vi "Predet_Ignite.vi"() -> (0 "Digital Waveform Graph":digitalwaveform[](graph), 3 "Error Out":errorcluster)   [LabVIEW 2017]
uses:
  <vilib>/DAQmx/write.llb/DAQmx Write (Digital 1D Wfm NChan NSamp).vi
  <vilib>/DAQmx/create/channels.llb/DAQmx Create Channel (DO-Digital Output).vi
  <vilib>/DAQmx/configure/timing.llb/DAQmx Timing (Sample Clock).vi
  <vilib>/Waveform/DTblOps.llb/DTbl Boolean Array to Digital.vi
  <vilib>/Waveform/DWDTOps.llb/DWDT Uncompress Digital.vi
  <vilib>/DAQmx/miscellaneous.llb/DAQmx Fill In Error Info.vi
  <resource>/objmgr/daqmx.rc
panel:
  in  "error in 2":errorcluster caption="error in"
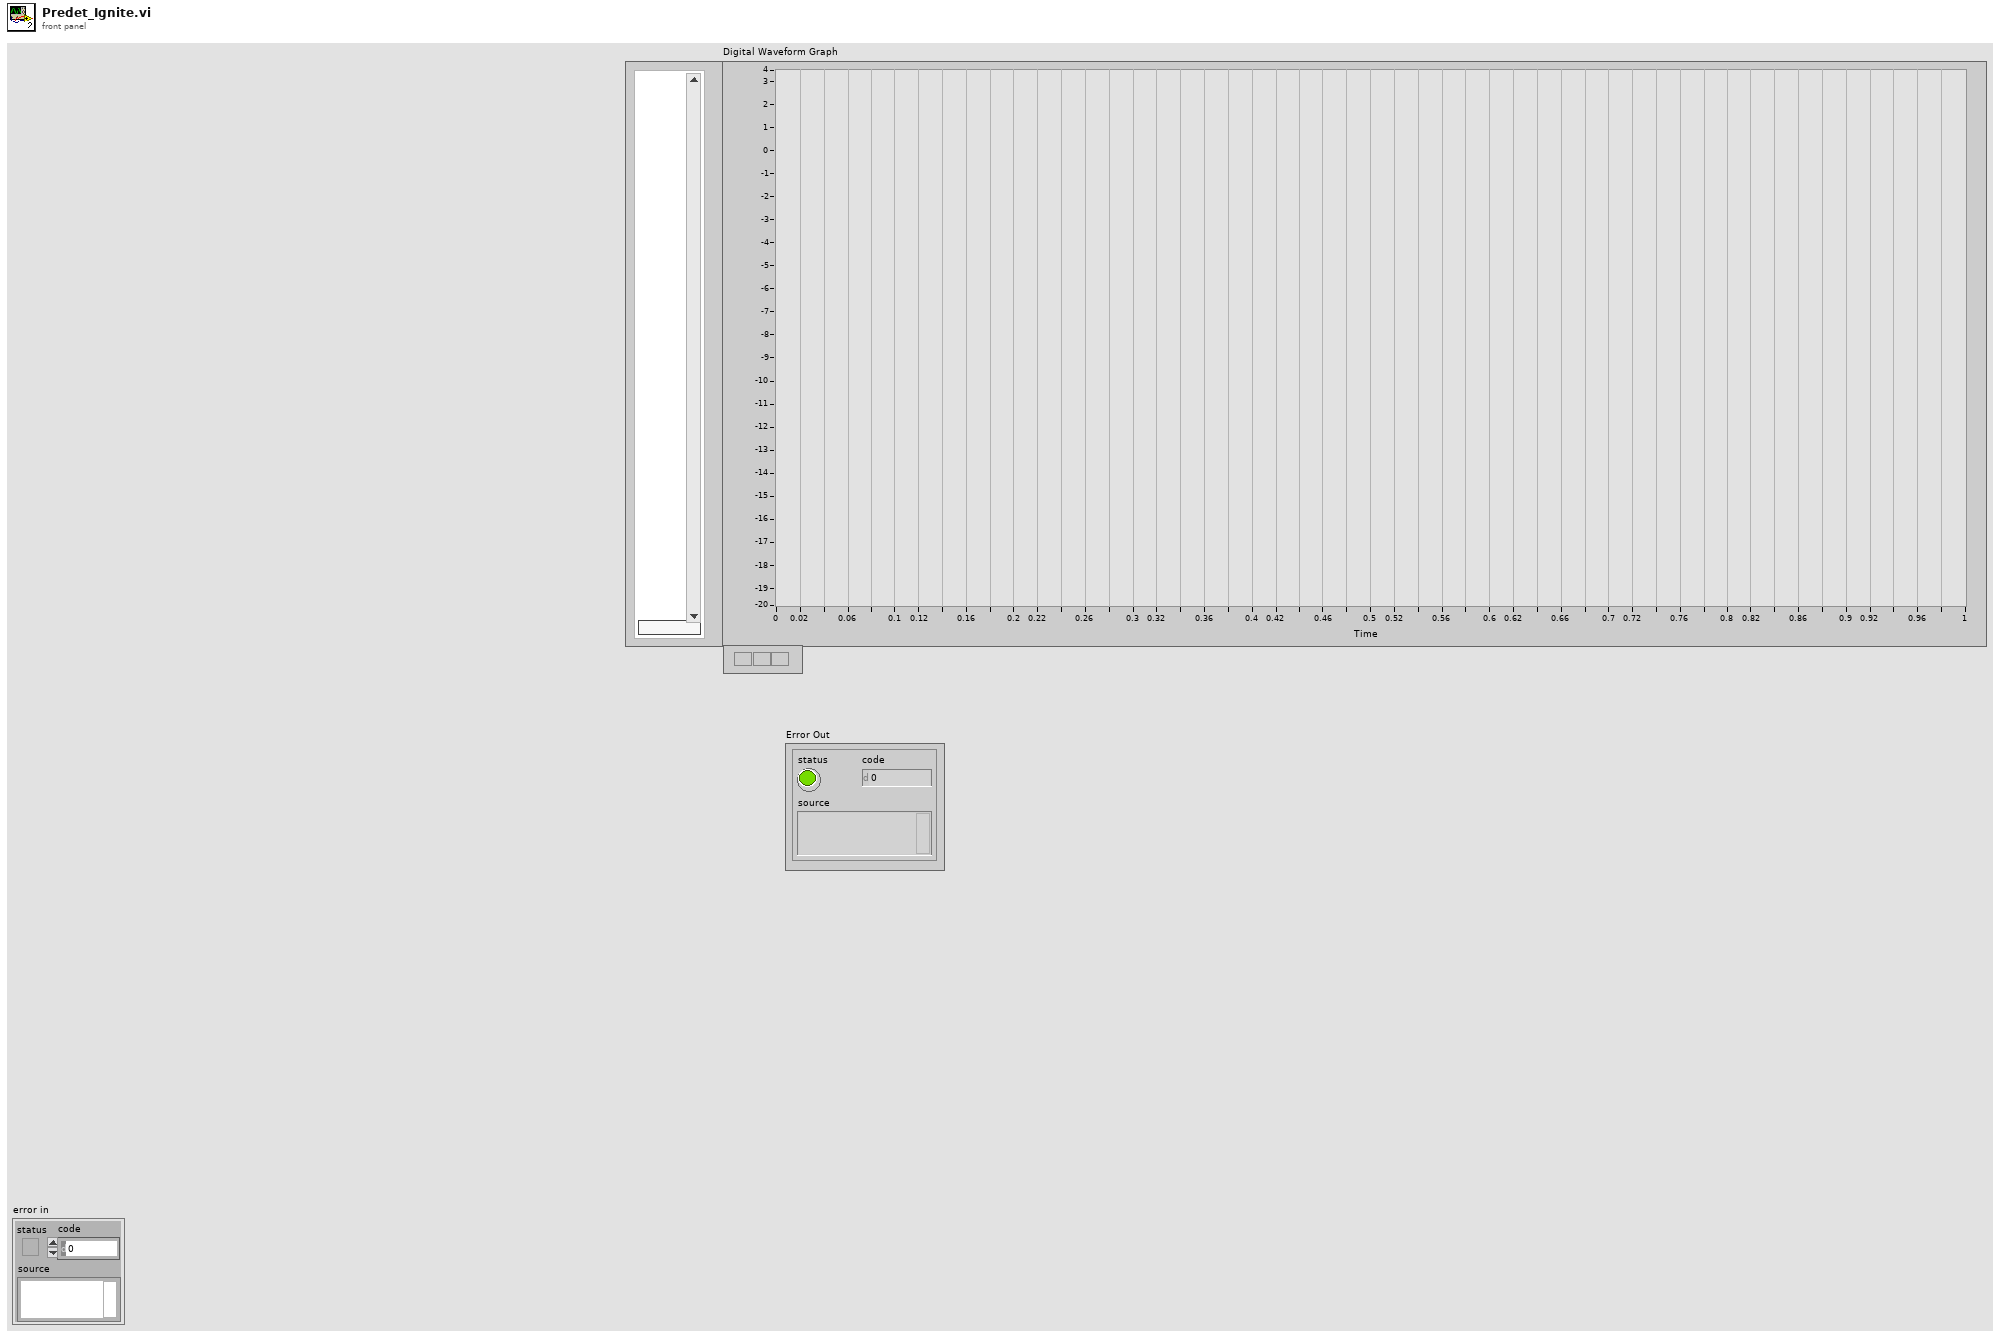
[diagram p1: front panel]
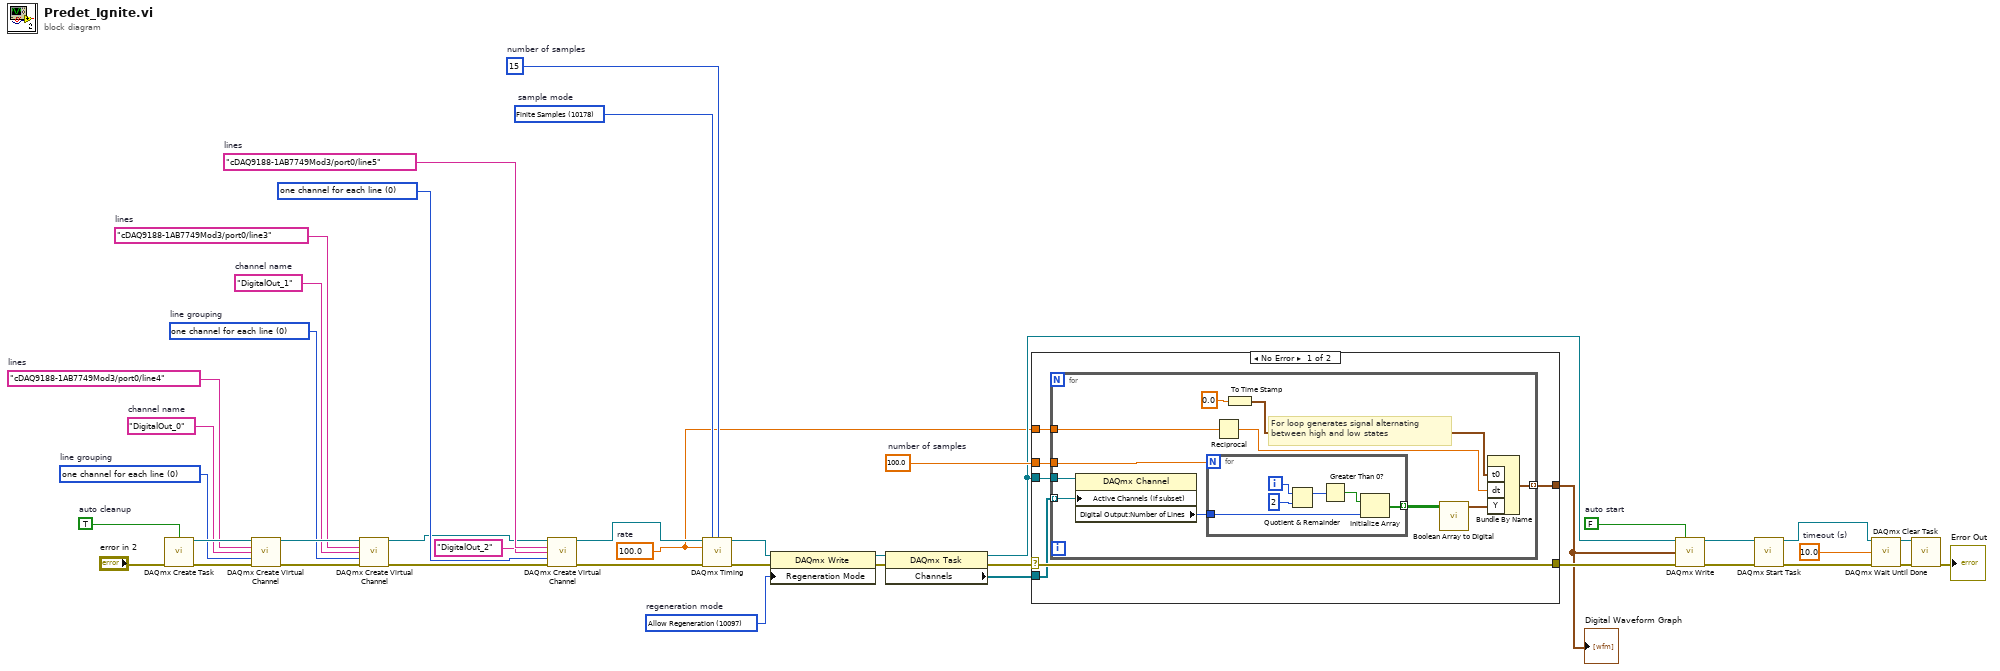
[diagram p0: block diagram]
diagram:
  w6 = "cDAQ9188-1AB7749Mod3/port0/line5"  # lines
  w7 = 0 items=["one channel for each line", "one channel for all lines"] ("line grouping")
  w13 = 10097 items=["Allow Regeneration"=10097, "Do Not Allow Regeneration"=10158]  # regeneration mode
  w15 = 10178 items=["Finite Samples"=10178, "Continuous Samples"=10123, "Hardware Timed Single Point"=12522]  # sample mode
  w16 = 15  # number of samples
  w1 = 100.0  # rate
  w19 = 0 items=["one channel for each line", "one channel for all lines"]  # line grouping
  w18 = "DigitalOut_1"  # channel name
  w20 = "cDAQ9188-1AB7749Mod3/port0/line3"  # lines
  w24 = 0 items=["one channel for each line", "one channel for all lines"]  # line grouping
  w23 = "DigitalOut_0"  # channel name
  w25 = "cDAQ9188-1AB7749Mod3/port0/line4"  # lines
  w27 = TRUE  # auto cleanup
  w35 = 10.0  # timeout (s)
  w32 = 100.0  # number of samples
  w42 = FALSE  # auto start
  n1 = call <vilib>:"DAQmx Create Task.vi"("auto cleanup"=w27, "error in"="error in 2") -> ("task out"=w26:refnum<k21>, "error out"=w28:errorcluster)  [unwired: 12 in]
  n2 = call-poly <vilib>:"DAQmx Create Virtual Channel.vi"("task in"=w26, "lines"=w25, "name to assign"=w23, "line grouping"=w24, "error in"=w28) -> ("task out"=w21:refnum<k21>, "error out"=w22:errorcluster)  [unwired: 9 in]
  n3 = call-poly <vilib>:"DAQmx Create Virtual Channel.vi"("task in"=w21, "lines"=w20, "name to assign"=w18, "line grouping"=w19, "error in"=w22) -> ("task out"=w4:refnum<k21>, "error out"=w9:errorcluster)  [unwired: 9 in]
  n4 = call-poly <vilib>:"DAQmx Create Virtual Channel.vi"("task in"=w4, "lines"=w6, "name to assign"="DigitalOut_2", "line grouping"=w7, "error in"=w9) -> ("task out"=w8:refnum<k21>, "error out"=w10:errorcluster)  [unwired: 9 in]
  n5 = call-poly <vilib>:"DAQmx Timing.vi"("task/channels in"=w8, "sample mode"=w15, "samples per channel"=w16, "rate"=w1, "error in"=w10) -> ("task out"=w14:refnum<k21>, "error out"=w17:errorcluster)  [unwired: 9 in]
  n6 = property class="DAQmx Write"(reference=w14, error in=w17, "Regeneration Mode"=w13) -> (reference out=w12:refnum<k21>, error out=w11:errorcluster)
  n7 = property class="DAQmx Task"(reference=w12, error in=w11) -> (reference out=w30:refnum<k21>, error out=w33:errorcluster, "Channels"=w34:refnum<k21>[])
  n8 = case shown="No Error" w33 {
    selector: w33 -> [w46 w66]
    tunnel: w1 -> [w48 _]
    tunnel: [w47 _] -> w3
    tunnel: [w46 w66] -> w31
    tunnel: w32 -> [w45 _]
    tunnel: w34 -> [w44 _]
    tunnel: w30 -> [w43 _]
    frame No Error {
      n9 = for {
        tunnel: w48 -> [w59]
        tunnel: [w54] -> w47 mode=indexing
        tunnel: w45 -> [w53]
        tunnel: w44 -> [w51] mode=indexing
        tunnel: w43 -> [w49]
        # "For loop generates signal alternating\nbetween high and low states"
        n10 = property class="DAQmx Channel"(reference=w49, "Active Channels (if subset)"=w51) -> ("Digital Output:Number of Lines"=w50:u32)  [unwired: 1 in, 2 out]
        n11 = for {
          N: w53 -> [_]
          tunnel: [w60] -> w52 mode=indexing
          tunnel: w50 -> [w61]
          i -> [w65]
          n12 = Quotient & Remainder(x=w65, y=2) -> (x-y*floor(x/y)=w63:i32)  [unwired: 1 out]
          n13 = Greater Than 0?(x=w63) -> (x > 0?=w62:bool)
          n14 = Initialize Array(w62, w61) -> (w60:bool[])
        }
        n15 = Reciprocal(x=w59) -> (1/x=w55:dbl)
        n16 = To Time Stamp(1:0.0) -> (0:w57:timestamp)
        n17 = call-poly <vilib>:"Boolean Array to Digital.vi"("boolean array"=w52) -> ("digital data"=w56:digitaldata)  [unwired: 3 in, 7 out]
        n18 = Bundle By Name("t0"=w57, "dt"=w55, "Y"=w56) -> (w54:digitalwaveform)  [unwired: 1 out]
      }
    }
    frame Error {
    }
  }
  "Digital Waveform Graph" <- w3
  n19 = call-poly <vilib>:"DAQmx Write.vi"("task/channels in"=w30, "auto start"=w42, "data"=w3, "error in"=w31) -> ("task out"=w38:refnum<k21>, "error out"=w37:errorcluster)  [unwired: 9 in, 1 out]
  n20 = call <vilib>:"DAQmx Start Task.vi"("task/channels in"=w38, "error in"=w37) -> ("task out"=w41:refnum<k21>, "error out"=w40:errorcluster)  [unwired: 12 in]
  n21 = call <vilib>:"DAQmx Wait Until Done.vi"("task/channels in"=w41, "timeout (sec)"=w35, "error in"=w40) -> ("task out"=w36:refnum<k21>, "error out"=w39:errorcluster)  [unwired: 11 in]
  n22 = call <vilib>:"DAQmx Clear Task.vi"("task in"=w36, "error in"=w39) -> ("error out"=→"Error Out":errorcluster)  [unwired: 13 in]
